vi "Global_DAQ.vi"() -> ()   [LabVIEW 2021]
panel:
  in  "Time Unit":T1(ring)=enum."MicroSecond"
  in  "Digital Sample  Frequency (Hz)":u32=10000000
  in  "Digital Sample Numbers":u32=20000000
  in  "Digital Data":u32[](array[numeric])
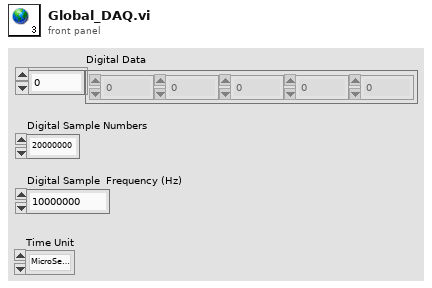
[diagram p1: front panel]
types:
  T1 = enum16{"NanoSecond", "MicroSecond", "MilliSecond"}
diagram:
